vi "ad next buffer.vi"(8 "error in (no error)":errorcluster, 9 "next":u32, 10 "buf":u32, 11 "adh":i32) -> (0 "error out":errorcluster, 1 "next out":u32, 3 "function return":i32)   [LabVIEW 2021, in "libad4.lvlib"]
doc: "LIBAD4 function: ad_next_buffer (int32_t adh, const void *buf, void **next);\n\nUpdates pointer to next buffer."
uses:
  <userlib>/libad4/libad4.lvlib
  <userlib>/libad4/libad4.dll
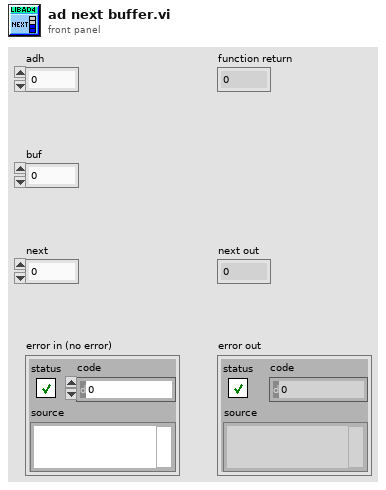
[diagram p1: front panel]
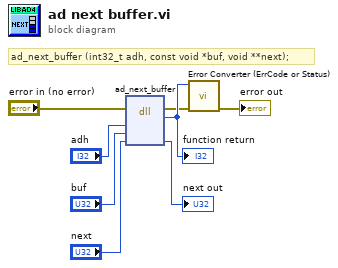
[diagram p0: block diagram]
diagram:
  # "ad_next_buffer (int32_t adh, const void *buf, void **next);"
  n1 = dll-call lib="C:/Program Files/National Instruments/LabVIEW 2021/user.lib/libad4/libad4.*" fn="ad_next_buffer"(error in="error in (no error)", "adh"="adh", "buf"="buf", "next"="next") -> (error out=w2:errorcluster, w8:i32, "next"=→"next out":u32)  [unwired: 4 in, 1 out]
  "function return" <- w8
  n2 = call <userlib>:"Error Converter (ErrCode or Status).vi"("error in (no error)"=w2, "error code"=w8) -> ("error out"=→"error out":errorcluster)  [unwired: 9 in]
